vi "GSP_Main.vi"() -> ()   [LabVIEW 2015]
uses:
  Systems/Cam_Focus/CF_drivercontrol.ctl
  Systems/Wavelength/wavelength_driver_actions.ctl
  Silvermax/Monitor/handler_actions.ctl
  Log/LogItem.ctl
  Systems/Coll_Focus/coll_actions.ctl
  Systems/Grating_Translation/GTdriveractions.ctl
  Systems/Primary Filter/f1driveractions.ctl
  Systems/Secondary Filter/f2driveractions.ctl
  Systems/Slit/slitactions.ctl
  Systems/TCS_Link/TCSLINK_handler_actions.ctl
  GUI/GUI_states.ctl
  Systems/Cam_Focus/GSP_CF_Global.vi
  Systems/Wavelength/GSP_Wavelength_Global.vi
  Systems/SIcamera_Control/GPS_Drivers/GPS_Driver_Global.vi
  GUI/GSP_GUI_global.vi
  Systems/Primary Filter/GSP_F1_Global.vi
  Systems/Grating_Translation/GSP_GT_Global.vi
  Systems/Slit/GSP_SLIT_Global.vi
  Systems/Secondary Filter/GSP_F2_Global.vi
panel:
  out "TCS Connected":u16(ring)
  out "Camera Focus":u16(ring)
  out "Collimator Focus":u16(ring)
  out "Camera/Grating":u16(ring)
  out "Grating Selection":u16(ring)
  out "Mask Assembly":u16(ring)
  out "Secondary Filter":u16(ring)
  out "Primary Filter":u16(ring)
  out "Shutter Open":u16(ring)=2
  out "Camera flex target":dbl
  in  "Active?":bool=TRUE
  out "Right":i32
  out "Left":i32
  out "AnimatedControl":u16(ring)
  out "Instrument Connected":u16(ring)
  out "Last Error":errorcluster
  # "Flexure   Compensation"
  # "Wavelength Subpanel"
  # "Grating Subpanel"
  # "Slit Subpanel"
  # "Camera Subpanel"
  # "Collimator Subpanel"
  # "F2 Subpanel"
  # "F1 Subpanel"
  # "TCS Link\nSubpanel"
  # "Camera Control Subpanel"
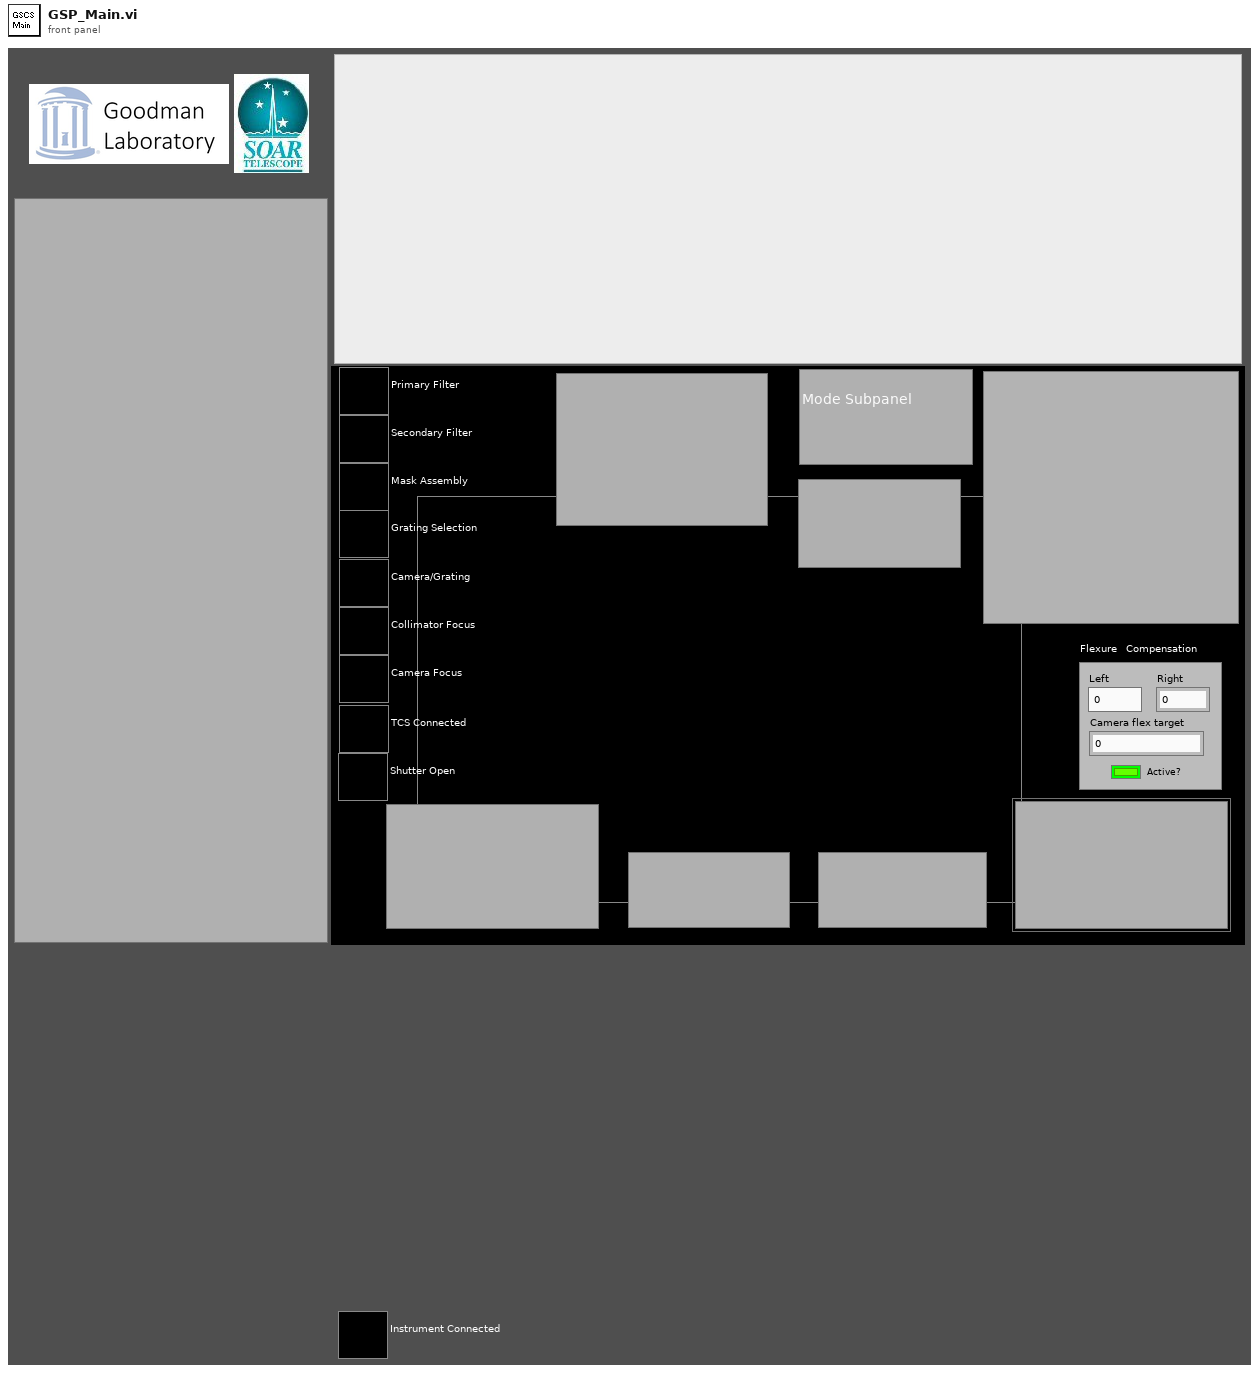
[diagram p1: front panel]
types:
  T1 = typedef "wavelength_driver_actions.ctl" = enum16{"Launch", "Flexure On", "Flexure Off", "Move", "Home", "Shutdown"}
  T2 = typedef "CF_drivercontrol.ctl" = enum16{"Launch", "Move", "Set Piezos", "Flexure On", "Flexure Off", "Home", "Shutdown"}
  T3 = typedef "handler_actions.ctl" = enum16{"Launch", "Shutdown All", "Shutdown"}
  T4 = enum16{"Launch", "Log", "Open", "Close", "Shutdown"}
  T5 = typedef "LogItem.ctl" = cluster{"error in (no error)":errorcluster, "Source":string, "Comment ":string}
  T6 = typedef "coll_actions.ctl" = enum16{"Launch", "Move", "Home", "Open Shutter", "Close Shutter", "Shutdown"}
  T7 = typedef "GTdriveractions.ctl" = enum16{"Launch", "INIT_CTL", "Move", "Home", "Shutdown"}
  T8 = typedef "f1driveractions.ctl" = enum16{"Launch", "INIT_CTL", "Home", "Move", "Shutdown"}
  T9 = typedef "f2driveractions.ctl" = enum16{"Launch", "INIT_CTL", "Home", "Move", "Shutdown"}
  T10 = typedef "slitactions.ctl" = enum16{"Launch", "INIT_CTL", "Restart", "Show", "Hide", "Home", "Move", "Rotate Only", "Shutdown"}
  T11 = typedef "TCSLINK_handler_actions.ctl" = enum16{"Launch", "Shutdown"}
  T12 = typedef "GUI_states.ctl" = enum16{"Logged Out", "Observer", "Operator", "Engineer"}
  T13 = cluster{"Primary Filter Names":string[], "Secondary Filter Names":string[], "Grating Names":string[], "Slit Mask Names":string[]}
  T14 = typedef "ThreadStates.ctl" = enum16{"Waiting", "Scripting", "Uninitialized", "Error"}
  T15 = cluster{"GT Thread state":T14, "Slit Thread State":T14, "F1 Thread State":T14, "F2 Thread State":T14, "Coll Thread State":T14, "CF Thread State":T14, "Wavelength Thread State":T14}
  T16 = cluster{"Grating#":i32, "Slit#":i32, "Primary Filter#":i32, "Secondary Filter#":i32, "Coll Position":i32, "Camera Focus":i32, "Camera Angle":dbl, "Grating Angle":dbl, "Coll Temp":dbl, "CF Temp\n":dbl, "Camera Target":dbl, "Grating Target":dbl, "WAVMODE":string, "Slit Hidden??":bool}
  T17 = cluster{"Init Primary Filter":bool, "Init Secondary Filter":bool, "Init Coll Focus":bool, "Init Camera Focus":bool, "Init Slit":bool, "Init Grating Trans":bool, "Init Wavelength":bool}
  T18 = cluster{"Primary Filter Names":string[], "Secondary Filter Names":string[], "Grating Names":string[], "Slit Mask Names":string[], "Standard Observing Modes":string[]}
  T19 = cluster{"F1_Name":string, "F2_Name":string, "Slit Name":string, "Grating Name":string, "Camera Target":dbl, "Grating Target":dbl, "Coll Position":i32, "Camera Focus":i32, string, string, string, string, "Flexure Active":bool, i32}
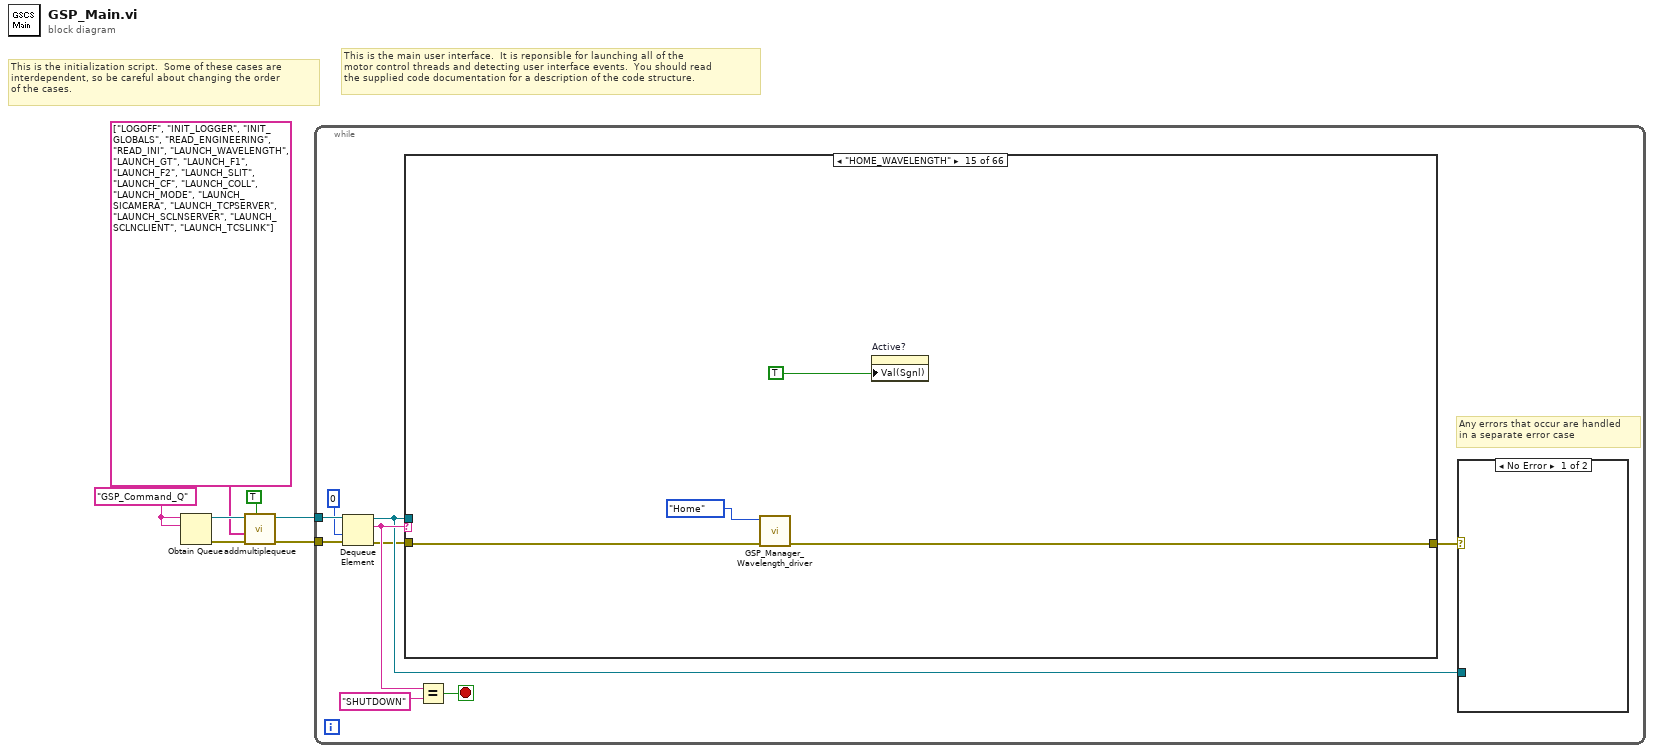
[diagram p0: block diagram]
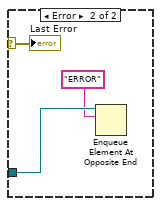
[diagram p2: hidden frame]
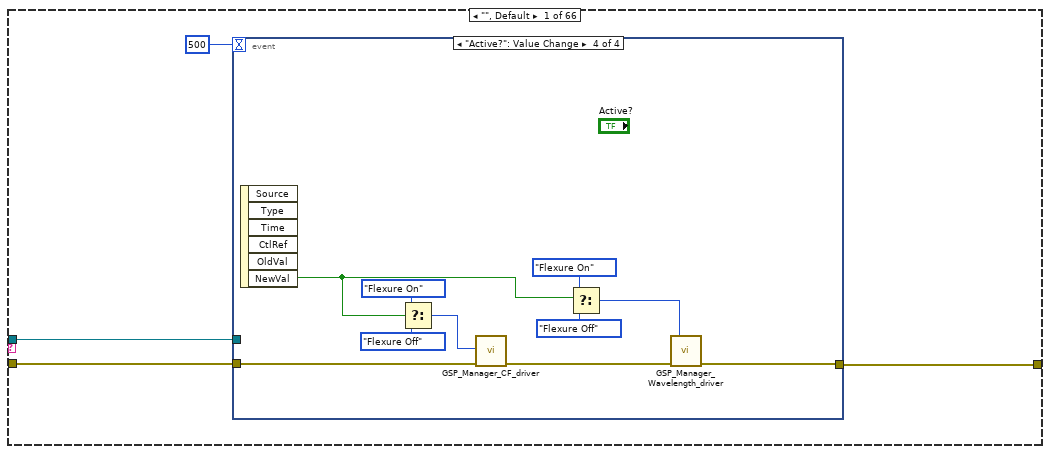
[diagram p3: hidden frame]
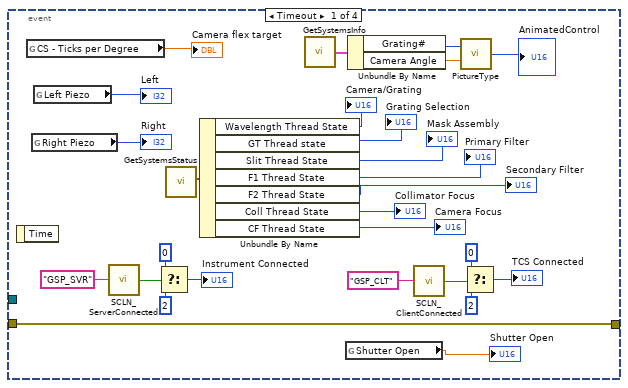
[diagram p4: hidden frame]
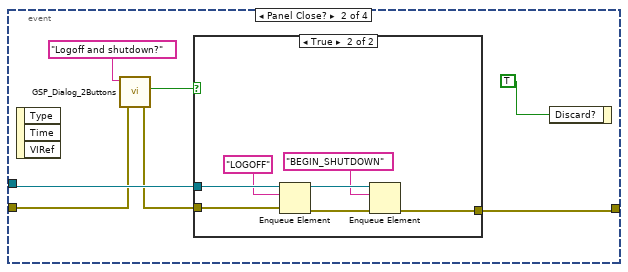
[diagram p5: hidden frame]
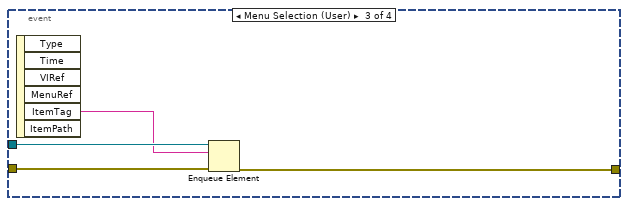
[diagram p7: hidden frame]
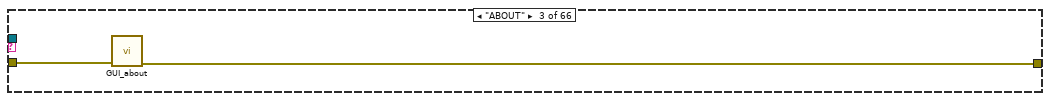
[diagram p9: hidden frame]
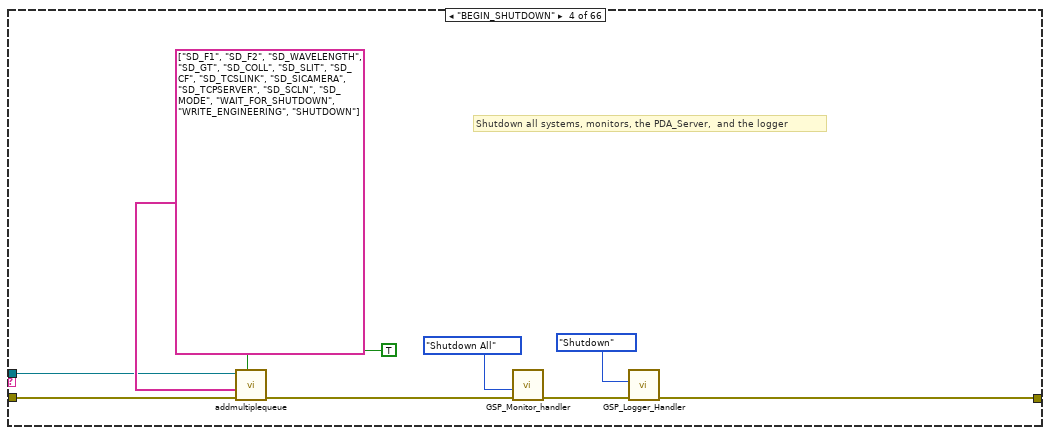
[diagram p10: hidden frame]
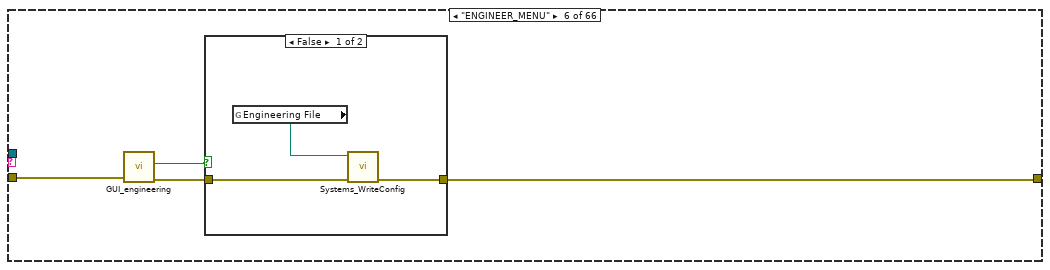
[diagram p12: hidden frame]
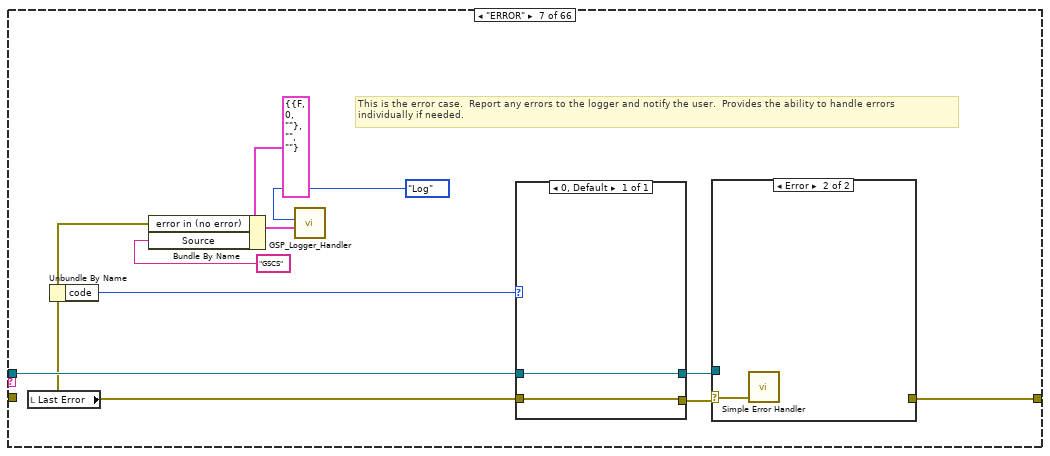
[diagram p14: hidden frame]
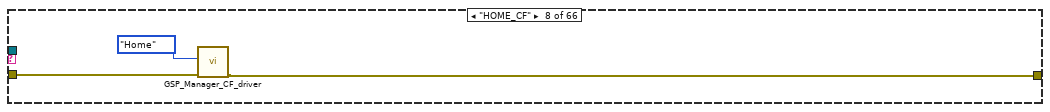
[diagram p16: hidden frame]
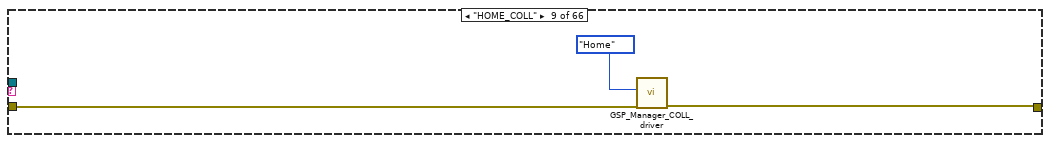
[diagram p17: hidden frame]
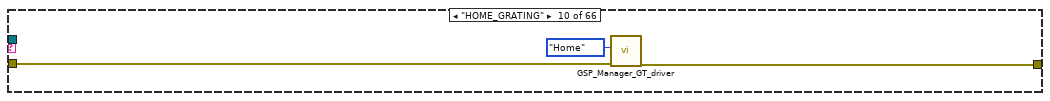
[diagram p18: hidden frame]
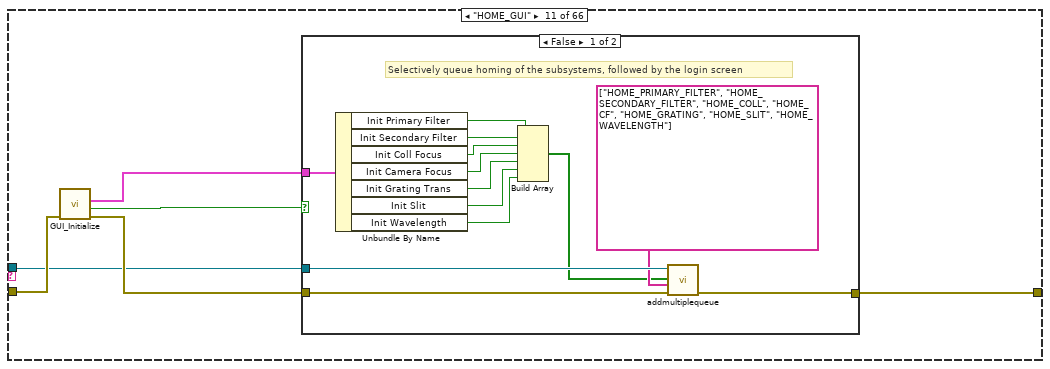
[diagram p19: hidden frame]
diagram:
  w7 = "GSP_Command_Q" ("name (unnamed)")
  # "This is the initialization script.  Some of these cases are\ninterdependent, so be careful about changing the order\nof the cases."
  # "This is the main user interface.  It is reponsible for launching all of the \nmotor control threads and detecting user interface events.  You should read \nthe supplied code documentation for a description of the code structure."
  n1 = Obtain Queue(name (unnamed)=w7, element data type=w7) -> (queue out=w3:refnum<queue>, error out=w5:errorcluster)  [unwired: 3 in, 1 out]
  n2 = call "addmultiplequeue.vi"("Add All (false)"=TRUE, "error in (no error)"=w5, "Strings to Add"=string[] ["LOGOFF", "INIT_LOGGER", "INIT_GLOBALS", "READ_ENGINEERING", "READ_INI", "LAUNCH_WAVELENGTH", "LAUNCH_GT", "LAUNCH_F1", "LAUNCH_F2", "LAUNCH_SLIT", "LAUNCH_CF", "LAUNCH_COLL", "LAUNCH_MODE", "LAUNCH_SICAMERA", "LAUNCH_TCPSERVER", "LAUNCH_SCLNSERVER", "LAUNCH_SCLNCLIENT", "LAUNCH_TCSLINK"], "queue"=w3) -> ("error out"=w1:errorcluster, "queue out"=w6:refnum<queue>)  [unwired: 3 in]
  n3 = while {
    tunnel: w1 -> [w15]
    tunnel: w6 -> [w16]
    stop <- w12 stop-if-true
    # "Any errors that occur are handled\nin a separate error case"
    n4 = Dequeue Element(queue=w16, timeout in ms (-1)=0, error in (no error)=w15) -> (queue out=w11:refnum<queue>, element=w14:string, error out=w9:errorcluster)  [unwired: 1 out]
    n5 = case shown="\"HOME_WAVELENGTH\"" w14 {
      tunnel: w11 -> [w23 _ _ w87 _ _ w108 _ _ _ w126 _ _ _ _ _ _ _ _ _ _ _ _ _ _ _ _ _ _ _ _ _ w267 w280 _ _ _ _ _ _ _ _ _ _ _ _ _ _ _ _ _ _ _ _ _ _ _ _ _ _ w425 _ _ _ _ _]
      tunnel: w9 -> [w22 w80 w82 w89 w92 w96 _ w117 w120 w123 w129 w146 w149 w152 w156 w165 w182 w197 w203 w208 w213 w218 w222 w228 w232 w237 w242 w248 w251 w254 w257 w258 w270 w283 w302 w308 w312 w319 w325 w332 w338 w344 w350 w354 w358 w365 w383 w386 w389 w391 w395 w398 w401 w404 w407 w409 w413 w416 _ w423 _ w432 w441 w445 w448 w449]
      tunnel: [w21 w80 w81 w83 w92 w93 w106 w115 w119 w122 w125 w145 w148 w151 w154 w158 w175 w196 w200 w204 w209 w215 w219 w225 w229 w235 w243 w246 w249 w252 w255 w261 w268 w279 w297 w303 w311 w315 w323 w328 w335 w341 w347 w352 w357 w365 w382 w385 w388 w392 w394 w397 w400 w403 w406 w408 w412 w415 _ w421 w424 w428 w436 w444 w447 _] -> w8
      frame "", Default {
        n6 = event shown="[3] \"Active?\": Value Change" {
          selector: _ -> [_ _ _ _]
          dyn-events: _ -> [_ _ _ _]
          timeout: 500 -> [_ _ _ _]
          tunnel: w23 -> [_ w56 w69 _]
          tunnel: [w43 w55 w66 w74] -> w21
          tunnel: w22 -> [w43 w53 w67 w79]
          event Timeout {
            n7 = event-data() -> ()  [unwired: 1 in, 1 out]
            n8 = global read "GSP_Wavelength_Global.vi" "CS - Ticks per Degree"() -> (→"Camera flex target":dbl)
            n9 = global read "GSP_CF_Global.vi" "Right Piezo"() -> (→"Right":i32)
            n10 = global read "GSP_CF_Global.vi" "Left Piezo"() -> (→"Left":i32)
            n11 = call "SCLN_ServerConnected.vi"("Server Name"="GSP_SVR" ("String")) -> ("Connected"=w31:bool)
            n12 = Select(t=u16 0, s=w31, f=u16 2) -> (s? t:f=→"Instrument Connected":u16)
            n13 = call "GetSystemsStatus.vi"() -> ("Thread States"=w42:T15)  [unwired: 4 in, 3 out]
            n14 = Unbundle By Name(w42) -> ("Wavelength Thread State"=→"Camera/Grating":T14, "GT Thread state"=→"Grating Selection":T14, "Slit Thread State"=→"Mask Assembly":T14, "F1 Thread State"=→"Primary Filter":T14, "F2 Thread State"=→"Secondary Filter":T14, "Coll Thread State"=→"Collimator Focus":T14, "CF Thread State"=→"Camera Focus":T14)
            n15 = call "GetSystemsInfo.vi"() -> ("Pos Info"=w47:T16)
            n16 = global read "GPS_Driver_Global.vi" "Shutter Open"() -> (→"Shutter Open":dbl)
            n17 = Unbundle By Name(w47) -> ("Grating#"=w46:i32, "Camera Angle"=w45:dbl)
            n18 = call "SCLN_ClientConnected.vi"("Server Name"="GSP_CLT" ("String")) -> ("Connected"=w27:bool)
            n19 = call "PictureType.vi"("Camera Angle"=w45, "Grating#"=w46) -> ("GS_picture_tab"=→"AnimatedControl":u16)
            n20 = Select(t=u16 0, s=w27, f=u16 2) -> (s? t:f=→"TCS Connected":u16)
          }
          event Panel Close? {
            n21 = event-data() -> ()  [unwired: 1 in, 3 out]
            n22 = call "GSP_Dialog_2Buttons.vi"("error in (no error)"=w53, "Message"="Logoff and shutdown?" ("message")) -> ("error out"=w52:errorcluster, "OK Button?"=w51:bool)  [unwired: 4 in]
            n23 = case shown="True" w51 {
              tunnel: w52 -> [w58 w64]
              tunnel: w56 -> [_ w65]
              tunnel: [w58 w61] -> w55
              frame False {
              }
              frame True {
                n24 = Enqueue Element(queue=w65, element="LOGOFF", error in (no error)=w64) -> (queue out=w63:refnum<queue>, error out=w62:errorcluster)  [unwired: 1 in, 1 out]
                n25 = Enqueue Element(queue=w63, element="BEGIN_SHUTDOWN", error in (no error)=w62) -> (error out=w61:errorcluster)  [unwired: 1 in, 2 out]
              }
            }
            n26 = event-data("Discard?"=TRUE) -> ()  [unwired: 1 in, 1 out]
          }
          event Menu Selection (User) {
            n27 = event-data() -> ("ItemTag"=w68:string)  [unwired: 1 in, 5 out]
            n28 = Enqueue Element(queue=w69, element=w68, error in (no error)=w67) -> (error out=w66:errorcluster)  [unwired: 1 in, 2 out]
          }
          event "Active?": Value Change {
            n29 = event-data() -> ("NewVal"=w71:bool)  [unwired: 1 in, 5 out]
            n30 = Select(t=CF_drivercontrol."Flexure On" ("Action"), s=w71, f=CF_drivercontrol."Flexure Off" ("Action")) -> (s? t:f=w76:T2)
            n31 = call "GSP_Manager_CF_driver.vi"("error in (no error)"=w79, "Action"=w76) -> ("error out"=w75:errorcluster)  [unwired: 5 in, 1 out]
            n32 = Select(t=wavelength_driver_actions."Flexure On" ("Action"), s=w71, f=wavelength_driver_actions."Flexure Off" ("Action")) -> (s? t:f=w70:T1)
            n33 = call "GSP_Manager_Wavelength_driver.vi"("error in (no error)"=w75, "Action"=w70) -> ("error out"=w74:errorcluster)  [unwired: 4 in, 1 out]
          }
        }
      }
      frame "REFRESH_CONTROLS" {
        # "This case addresses a bug in remote panel builds.  Forces\na refresh of the control.disabled property for controls on the remote\npanel"
      }
      frame "ABOUT" {
        n34 = call "GUI_about.vi"("error in (no error)"=w82) -> ("error out"=w81:errorcluster)  [unwired: 6 in]
      }
      frame "BEGIN_SHUTDOWN" {
        # "Shutdown all systems, monitors, the PDA_Server,  and the logger"
        n35 = call "addmultiplequeue.vi"("Add All (false)"=TRUE, "error in (no error)"=w89, "Strings to Add"=string[] ["SD_F1", "SD_F2", "SD_WAVELENGTH", "SD_GT", "SD_COLL", "SD_SLIT", "SD_CF", "SD_TCSLINK", "SD_SICAMERA", "SD_TCPSERVER", "SD_SCLN", "SD_MODE", "WAIT_FOR_SHUTDOWN", "WRITE_ENGINEERING", "SHUTDOWN"], "queue"=w87) -> ("error out"=w88:errorcluster)  [unwired: 3 in, 1 out]
        n36 = call "GSP_Monitor_handler.vi"("error in (no error)"=w88, "Action"=handler_actions."Shutdown All") -> ("error out"=w86:errorcluster)  [unwired: 5 in, 1 out]
        n37 = call "GSP_Logger_Handler.vi"("error in (no error)"=w86, "Actions"=T4."Shutdown") -> ("error out"=w83:errorcluster)  [unwired: 5 in]
      }
      frame "DOCUMENTATION" {
      }
      frame "ENGINEER_MENU" {
        n38 = call "GUI_engineering.vi"("error in (no error)"=w96) -> ("error out"=w95:errorcluster, "Canceled?"=w94:bool)  [unwired: 5 in]
        n39 = case shown="False" w94 {
          tunnel: w95 -> [w99 w100]
          tunnel: [w98 w100] -> w93
          frame False {
            n40 = global read "GSP_GUI_global.vi" "Engineering File"() -> (w97:path)
            n41 = call "Systems_WriteConfig.vi"("error in (no error)"=w99, "configuration file path"=w97) -> ("error out"=w98:errorcluster)  [unwired: 5 in]
          }
          frame True {
          }
        }
      }
      frame "ERROR" {
        # "This is the error case.  Report any errors to the logger and notify the user.  Provides the ability to handle errors\nindividually if needed."
        n42 = local read "Last Error"() -> (w102:errorcluster)
        n43 = Unbundle By Name(w102) -> ("code"=w110:i32)
        n44 = Bundle By Name(cluster=T5 {"error in (no error)"={"status"=FALSE, "code"=0, "source"=""}, "Source"="", "Comment "=""} ("Log"), "error in (no error)"=w102, "Source"="GSCS") -> (w103:T5)
        n45 = call "GSP_Logger_Handler.vi"("Log"=w103, "Actions"=T4."Log") -> ()  [unwired: 5 in, 1 out]
        n46 = case shown="0, Default" w110 {
          tunnel: w102 -> [w114]
          tunnel: [w114] -> w109
          tunnel: w108 -> [w113]
          tunnel: [w113] -> w107
          frame 0, Default {
          }
        }
        n47 = case shown="Error" w109 {
          selector: w109 -> [w111 w112]
          tunnel: [w111 _] -> w106
          tunnel: w107 -> [_ _]
          frame No Error {
          }
          frame Error {
            n48 = call <vilib>:"Simple Error Handler.vi"("error in (no error)"=w112) -> ()  [unwired: 4 in, 5 out]
          }
        }
      }
      frame "HOME_CF" {
        n49 = call "GSP_Manager_CF_driver.vi"("error in (no error)"=w117, "Action"=CF_drivercontrol."Home") -> ("error out"=w115:errorcluster)  [unwired: 5 in, 1 out]
      }
      frame "HOME_COLL" {
        n50 = call "GSP_Manager_COLL_driver.vi"("error in (no error)"=w120, "Action"=coll_actions."Home") -> ("error out"=w119:errorcluster)  [unwired: 4 in, 1 out]
      }
      frame "HOME_GRATING" {
        n51 = call "GSP_Manager_GT_driver.vi"("error in (no error)"=w123, "Action"=GTdriveractions."Home") -> ("error out"=w122:errorcluster)  [unwired: 4 in, 1 out]
      }
      frame "HOME_GUI" {
        n52 = call "GUI_Initialize.vi"("error in (no error)"=w129) -> ("error out"=w128:errorcluster, "Canceled?"=w127:bool, "Initialize Out"=w124:T17)  [unwired: 4 in]
        n53 = case shown="False" w127 {
          tunnel: w128 -> [w141 w143]
          tunnel: w126 -> [w140 _]
          tunnel: [w130 w143] -> w125
          tunnel: w124 -> [w142 _]
          frame False {
            # "Selectively queue homing of the subsystems, followed by the login screen"
            n54 = Unbundle By Name(w142) -> ("Init Primary Filter"=w137:bool, "Init Secondary Filter"=w131:bool, "Init Coll Focus"=w136:bool, "Init Camera Focus"=w135:bool, "Init Grating Trans"=w134:bool, "Init Slit"=w133:bool, "Init Wavelength"=w132:bool)
            n55 = Build Array(w137, w131, w136, w135, w134, w133, w132) -> (w138:bool[])
            n56 = call "addmultiplequeue.vi"("error in (no error)"=w141, "Strings to Add"=string[] ["HOME_PRIMARY_FILTER", "HOME_SECONDARY_FILTER", "HOME_COLL", "HOME_CF", "HOME_GRATING", "HOME_SLIT", "HOME_WAVELENGTH"], "Add String?"=w138, "queue"=w140) -> ("error out"=w130:errorcluster)  [unwired: 3 in, 1 out]
          }
          frame True {
          }
        }
      }
      frame "HOME_PRIMARY_FILTER" {
        n57 = call "GSP_Manager_F1_driver.vi"("error in (no error)"=w146, "Action"=f1driveractions."Home") -> ("error out"=w145:errorcluster)  [unwired: 4 in, 1 out]
      }
      frame "HOME_SECONDARY_FILTER" {
        n58 = call "GSP_Manager_F2_driver.vi"("error in (no error)"=w149, "Action"=f2driveractions."Home") -> ("error out"=w148:errorcluster)  [unwired: 4 in, 1 out]
      }
      frame "HOME_SLIT" {
        n59 = call "GSP_Manager_Slit_driver.vi"("error in (no error)"=w152, "Action"=slitactions."Home") -> ("error out"=w151:errorcluster)  [unwired: 4 in, 1 out]
      }
      frame "HOME_WAVELENGTH" {
        n60 = call "GSP_Manager_Wavelength_driver.vi"("error in (no error)"=w156, "Action"=wavelength_driver_actions."Home") -> ("error out"=w154:errorcluster)  [unwired: 4 in, 1 out]
        n61 = property on="Active?" class="Bool (strict)"("Val(Sgnl)"=TRUE) -> ()  [unwired: 2 in, 2 out]
      }
      frame "INIT_CONTROLS" {
        n62 = call "GSP_Manager_F1_driver.vi"("error in (no error)"=w165, "Action"=f1driveractions."INIT_CTL") -> ("error out"=w163:errorcluster)  [unwired: 4 in, 1 out]
        n63 = call "GSP_Manager_F2_driver.vi"("error in (no error)"=w163, "Action"=f2driveractions."INIT_CTL") -> ("error out"=w161:errorcluster)  [unwired: 4 in, 1 out]
        n64 = call "GSP_Manager_Slit_driver.vi"("error in (no error)"=w161, "Action"=slitactions."INIT_CTL") -> ("error out"=w159:errorcluster)  [unwired: 4 in, 1 out]
        n65 = call "GSP_Manager_GT_driver.vi"("error in (no error)"=w159, "Action"=GTdriveractions."INIT_CTL") -> ("error out"=w158:errorcluster)  [unwired: 4 in, 1 out]
      }
      frame "INIT_GLOBALS" {
        w169 = path "\\\\SHERMAN-PC\\Config"
        # "Detects wether this is a build or development"
        # "Initialize all of the global file paths, detecting wether you are in a build\nor development environment."
        # "Initialize the Silvermax serial port and reboot all of the motors using the group ID"
        n66 = call "gsp_silvermax_setup.vi"("error in (no error)"=w182, "Timeout (1000 ms)"=u32 100, "VISA resource name"=refnum<visa-resource-name> "COM1") -> ("error out"=w175:errorcluster)  [unwired: 4 in]
        n67 = Current VI's Path() -> (path=w187:path)
        n68 = Strip Path(path=w187) -> (stripped path=w166:path, name=w167:string)
        n69 = local write "Active?"(FALSE) -> ()
        n70 = Match Pattern(string=w167, regular expression=".exe") -> (offset past match=w191:i32)  [unwired: 1 in, 3 out]
        n71 = case shown="0, Default" w191 {
          tunnel: w166 -> [w194 w195]
          tunnel: [w194 w195] -> w171
          tunnel: w167 -> [_ _]
          frame 0, Default {
          }
          frame -1 {
          }
        }
        n72 = Build Path(base path=w169, name or relative path="observing_modes.ini") -> (appended path=w173:path)
        n73 = Build Path(base path=w169, name or relative path="engineering.ini") -> (appended path=w193:path)
        n74 = global write "GSP_GUI_global.vi" "Standard Observing Modes File"(w173) -> ()
        n75 = global write "GSP_GUI_global.vi" "Engineering File"(w193) -> ()
        n76 = Build Path(base path=w169, name or relative path="masks.ini") -> (appended path=w178:path)
        n77 = Build Path(base path=w169, name or relative path="filters.ini") -> (appended path=w179:path)
        n78 = Build Path(base path=w169, name or relative path="gratings.ini") -> (appended path=w185:path)
        n79 = Build Path(base path=w169, name or relative path="masterconfig.ini") -> (appended path=w170:path)
        n80 = Build Path(base path=w171, name or relative path="users.ini") -> (appended path=w177:path)
        n81 = Build Path(base path=w171, name or relative path="Users") -> (appended path=w189:path)
        n82 = global write "GSP_GUI_global.vi" "Configuration File"(w170) -> ()
        n83 = global write "GSP_GUI_global.vi" "UserFile"(w177) -> ()
        n84 = global write "GSP_GUI_global.vi" "Filter File"(w179) -> ()
        n85 = global write "GSP_GUI_global.vi" "Slit File"(w178) -> ()
        n86 = global write "GSP_GUI_global.vi" "Grating File"(w185) -> ()
        n87 = global write "GSP_GUI_global.vi" "UserPath"(w189) -> ()
      }
      frame "INIT_LOGGER" {
        n88 = call "GSP_Logger_Handler.vi"("error in (no error)"=w197, "Actions"=T4."Launch") -> ("error out"=w196:errorcluster)  [unwired: 5 in]
      }
      frame "LAUNCH_WAVELENGTH" {
        # "Motor manager threads are launched by supplying control references to the controls that threads will update.  This case launches\nthe collimator thread.  Events on the controls are still detected in the main interface and relayed to the manager threads by using the\ninterface below with the appropriate action."
        n89 = call "GSP_Manager_Wavelength_driver.vi"("error in (no error)"=w203, "Action"=wavelength_driver_actions."Launch") -> ("error out"=w201:errorcluster, "VI reference (launch only)"=w199:refnum<vi>)  [unwired: 4 in]
        n90 = invoke on="Camera/Grating Angles" class="SubPanel" method="Insert VI"(error in=w201, "VI Ref"=w199) -> (error out=w200:errorcluster)  [unwired: 2 in, 3 out]
      }
      frame "LAUNCH_COLL" {
        n91 = call "GSP_Manager_COLL_driver.vi"("error in (no error)"=w208, "Action"=coll_actions."Launch") -> ("error out"=w206:errorcluster, "reference out (launch only)"=w205:refnum<vi>)  [unwired: 4 in]
        n92 = invoke on="Collimator Subpanel" class="SubPanel" method="Insert VI"(error in=w206, "VI Ref"=w205) -> (error out=w204:errorcluster)  [unwired: 2 in, 3 out]
      }
      frame "LAUNCH_CF" {
        n93 = call "GSP_Manager_CF_driver.vi"("error in (no error)"=w213, "Action"=CF_drivercontrol."Launch") -> ("error out"=w211:errorcluster, "reference out (launch only)"=w210:refnum<vi>)  [unwired: 5 in]
        n94 = invoke on="Camera Subpanel" class="SubPanel" method="Insert VI"(error in=w211, "VI Ref"=w210) -> (error out=w209:errorcluster)  [unwired: 2 in, 3 out]
      }
      frame "LAUNCH_F1" {
        n95 = call "GSP_Manager_F1_driver.vi"("error in (no error)"=w218, "Action"=f1driveractions."Launch") -> ("error out"=w217:errorcluster, "reference out (launch only)"=w216:refnum<vi>)  [unwired: 4 in]
        n96 = invoke on="F1 Subpanel" class="SubPanel" method="Insert VI"(error in=w217, "VI Ref"=w216) -> (error out=w215:errorcluster)  [unwired: 2 in, 3 out]
      }
      frame "LAUNCH_F2" {
        n97 = call "GSP_Manager_F2_driver.vi"("error in (no error)"=w222, "Action"=f2driveractions."Launch") -> ("error out"=w221:errorcluster, "reference out (launch only)"=w220:refnum<vi>)  [unwired: 4 in]
        n98 = invoke on="F1 Subpanel" class="SubPanel" method="Insert VI"(error in=w221, "VI Ref"=w220) -> (error out=w219:errorcluster)  [unwired: 2 in, 3 out]
      }
      frame "LAUNCH_GT" {
        n99 = call "GSP_Manager_GT_driver.vi"("error in (no error)"=w228, "Action"=GTdriveractions."Launch") -> ("error out"=w227:errorcluster, "reference out (launch only)"=w226:refnum<vi>)  [unwired: 4 in]
        n100 = invoke on="Grating Subpanel" class="SubPanel" method="Insert VI"(error in=w227, "VI Ref"=w226) -> (error out=w225:errorcluster)  [unwired: 2 in, 3 out]
      }
      frame "LAUNCH_SLIT" {
        n101 = call "GSP_Manager_Slit_driver.vi"("error in (no error)"=w232, "Action"=slitactions."Launch") -> ("error out"=w231:errorcluster, "reference out (launch only)"=w230:refnum<vi>)  [unwired: 4 in]
        n102 = invoke on="Slit Subpanel" class="SubPanel" method="Insert VI"(error in=w231, "VI Ref"=w230) -> (error out=w229:errorcluster)  [unwired: 2 in, 3 out]
      }
      frame "LAUNCH_TCSLINK" {
        n103 = call "GSP_Manager_TCSLINK_handler.vi"("error in (no error)"=w237, "Actions"=TCSLINK_handler_actions."Launch") -> ("error out"=w236:errorcluster, "reference out (launch only)"=w234:refnum<vi>)  [unwired: 4 in]
        n104 = invoke on="TCS_SubPanel" class="SubPanel" method="Insert VI"(error in=w236, "VI Ref"=w234) -> (error out=w235:errorcluster)  [unwired: 2 in, 3 out]
      }
      frame "LAUNCH_SICAMERA" {
        n105 = call "SIcamera_Driver.vi"("error in (no error)"=w242, "Action"=enum16{"Launch", "Shutdown"}."Launch") -> ("error out"=w239:errorcluster, "reference out (launch only)"=w240:refnum<vi>)  [unwired: 4 in]
        n106 = invoke on="SIcamera Control Panel" class="SubPanel" method="Insert VI"(error in=w239, "VI Ref"=w240) -> (error out=w243:errorcluster)  [unwired: 2 in, 3 out]
      }
      frame "LAUNCH_MODE" {
        n107 = call "Mode_driver.vi"("error in (no error)"=w248, "Action"=enum16{"Launch", "Shutdown"}."Launch") -> ("error out"=w247:errorcluster, "reference out (launch only)"=w244:refnum<vi>)  [unwired: 4 in]
        n108 = invoke on="Mode Subpanel" class="SubPanel" method="Insert VI"(error in=w247, "VI Ref"=w244) -> (error out=w246:errorcluster)  [unwired: 2 in, 3 out]
      }
      frame "LAUNCH_TCPSERVER" {
        n109 = call "TCPServer_driver.vi"("error in (no error)"=w251, "Action"=enum16{"Launch", "Shutdown"}."Launch") -> ("error out"=w249:errorcluster)  [unwired: 5 in]
      }
      frame "LAUNCH_SCLNSERVER" {
        n110 = call "GSP_Manager_SCLNServer_Handler.vi"("error in (no error)"=w254, "Actions"=TCSLINK_handler_actions."Launch") -> ("error out"=w252:errorcluster)  [unwired: 4 in, 1 out]
      }
      frame "LAUNCH_SCLNCLIENT" {
        n111 = call "GSP_Manager_SCLNClient_Handler.vi"("error in (no error)"=w257, "Actions"=TCSLINK_handler_actions."Launch") -> ("error out"=w255:errorcluster)  [unwired: 4 in, 1 out]
      }
      frame "LOGOFF" {
        # "Set the interface to a Logged Off mode"
        n112 = global write "GSP_GUI_global.vi" "Current User"("NO USER" ("Current User")) -> ()
        n113 = global write "GSP_GUI_global.vi" "User Type"(i8 0 ("User Type")) -> ()
        n114 = Current VI's Menubar() -> (w263:refnum<k9>)
        n115 = call "GSP_setmenu.vi"("error in (no error)"=w258, "GUI States"=GUI_states."Logged Out", "menubar"=w263) -> ("error out"=w261:errorcluster)  [unwired: 4 in]
      }
      frame "LOGON" {
        n116 = global read "GSP_GUI_global.vi" "UserFile"() -> (w264:path)
        n117 = call "GSP_GUI_user.vi"("error in"=w270, "User File"=w264) -> ("error out"=w269:errorcluster, "User Type"=w265:T12, "Canceled?"=w266:bool)  [unwired: 3 in]
        n118 = case shown="False" w266 {
          tunnel: w269 -> [w271 w275]
          tunnel: [w272 w275] -> w268
          tunnel: w267 -> [_ _]
          tunnel: w265 -> [w273 _]
          frame False {
            n119 = Current VI's Menubar() -> (w274:refnum<k9>)
            n120 = call "GSP_setmenu.vi"("error in (no error)"=w271, "GUI States"=w273, "menubar"=w274) -> ("error out"=w272:errorcluster)  [unwired: 4 in]
          }
          frame True {
          }
        }
      }
      frame "MASTER_CONFIG_GUI" {
        # "Open the Configuration Manager. If the user makes changes to the configuration file, reload the file and update the controls."
        n121 = global read "GSP_GUI_global.vi" "Filter File"() -> (w277:path)
        n122 = global read "GSP_GUI_global.vi" "Slit File"() -> (w276:path)
        n123 = global read "GSP_GUI_global.vi" "Grating File"() -> (w278:path)
        n124 = call "GSP_MasterConfiguration.vi"("error in (no error)"=w283, "Slit File"=w276, "Filter File"=w277, "grating file"=w278) -> ("error out"=w281:errorcluster, "Changes Made?"=w282:bool)  [unwired: 3 in]
        n125 = case shown="True" w282 {
          tunnel: w281 -> [w284 w293]
          tunnel: w280 -> [_ w294]
          tunnel: [w284 w296] -> w279
          frame False {
          }
          frame True {
            n126 = global read "GSP_GUI_global.vi" "Secondary Filter Names"() -> (w288:string[])
            n127 = global read "GSP_GUI_global.vi" "Primary Filter Names"() -> (w289:string[])
            n128 = global read "GSP_GUI_global.vi" "Grating Names"() -> (w287:string[])
            n129 = global read "GSP_GUI_global.vi" "Slit Mask Names"() -> (w286:string[])
            n130 = Bundle By Name(cluster=T13 {"Primary Filter Names"=[], "Secondary Filter Names"=[], "Grating Names"=[], "Slit Mask Names"=[]} ("Present Configuration"), "Primary Filter Names"=w289, "Secondary Filter Names"=w288, "Grating Names"=w287, "Slit Mask Names"=w286) -> (w285:T13)
            n131 = global read "GSP_GUI_global.vi" "Configuration File"() -> (w291:path)
            n132 = call "Write_Master_Config.vi"("error in (no error)"=w293, "Present Configuration"=w285, "configuration file path"=w291) -> ("error out"=w292:errorcluster)  [unwired: 4 in]
            n133 = Enqueue Element(queue=w294, element="INIT_CONTROLS", error in (no error)=w292) -> (error out=w296:errorcluster)  [unwired: 1 in, 2 out]
          }
        }
      }
      frame "MONITOR_COLL" {
        w299 = u16 1 items=["External", "Internal"] ("Mode")
        # "This is an example of how to launch a motor monitor and open the front panel"
        n134 = call "GSP_Monitor_handler.vi"("Mode"=w299, "error in (no error)"=w302, "Action"=handler_actions."Launch", "Motor#"=u8 40, "Monitor Name"="Collimator Focus") -> ("error out"=w297:errorcluster)  [unwired: 2 in, 1 out]
      }
      frame "MONITOR_CF" {
        w305 = u16 1 items=["External", "Internal"] ("Mode")
        # "This is an example of how to launch a motor monitor and open the front panel"
        n135 = call "GSP_Monitor_handler.vi"("Mode"=w305, "error in (no error)"=w308, "Action"=handler_actions."Launch", "Motor#"=u8 46, "Monitor Name"="Camera Focus") -> ("error out"=w303:errorcluster)  [unwired: 2 in, 1 out]
      }
      frame "MONITOR_CS" {
        w310 = u16 0 items=["External", "Internal"] ("Mode")
        n136 = call "GSP_Monitor_handler.vi"("Mode"=w310, "error in (no error)"=w312, "Action"=handler_actions."Launch", "Motor#"=u8 45, "Monitor Name"="Camera Stage") -> ("error out"=w311:errorcluster)  [unwired: 2 in, 1 out]
      }
      frame "MONITOR_F1" {
        w317 = u16 1 items=["External", "Internal"] ("Mode")
        n137 = call "GSP_Monitor_handler.vi"("Mode"=w317, "error in (no error)"=w319, "Action"=handler_actions."Launch", "Motor#"=u8 47, "Monitor Name"="Primary Filter Wheel") -> ("error out"=w315:errorcluster)  [unwired: 2 in, 1 out]
      }
      frame "MONITOR_F2" {
        w322 = u16 1 items=["External", "Internal"] ("Mode")
        n138 = call "GSP_Monitor_handler.vi"("Mode"=w322, "error in (no error)"=w325, "Action"=handler_actions."Launch", "Motor#"=u8 48, "Monitor Name"="Secondary Filter Wheel") -> ("error out"=w323:errorcluster)  [unwired: 2 in, 1 out]
      }
      frame "MONITOR_GS" {
        w329 = u16 0 items=["External", "Internal"] ("Mode")
        n139 = call "GSP_Monitor_handler.vi"("Mode"=w329, "error in (no error)"=w332, "Action"=handler_actions."Launch", "Motor#"=u8 43, "Monitor Name"="Grating Stage") -> ("error out"=w328:errorcluster)  [unwired: 2 in, 1 out]
      }
      frame "MONITOR_GT" {
        w334 = u16 1 items=["External", "Internal"] ("Mode")
        n140 = call "GSP_Monitor_handler.vi"("Mode"=w334, "error in (no error)"=w338, "Action"=handler_actions."Launch", "Motor#"=u8 44, "Monitor Name"="Grating Translation") -> ("error out"=w335:errorcluster)  [unwired: 2 in, 1 out]
      }
      frame "MONITOR_SLIT_ROT" {
        w339 = u16 1 items=["External", "Internal"] ("Mode")
        n141 = call "GSP_Monitor_handler.vi"("Mode"=w339, "error in (no error)"=w344, "Action"=handler_actions."Launch", "Motor#"=u8 41, "Monitor Name"="Slit Rotation") -> ("error out"=w341:errorcluster)  [unwired: 2 in, 1 out]
      }
      frame "MONITOR_SLIT_TRANS" {
        w346 = u16 1 items=["External", "Internal"] ("Mode")
        n142 = call "GSP_Monitor_handler.vi"("Mode"=w346, "error in (no error)"=w350, "Action"=handler_actions."Launch", "Motor#"=u8 42, "Monitor Name"="Slit Translation") -> ("error out"=w347:errorcluster)  [unwired: 2 in, 1 out]
      }
      frame "READ_ENGINEERING" {
        # "Read the engineering file.  This loads all of the motor manager global variables with the appropriate values."
        n143 = global read "GSP_GUI_global.vi" "Engineering File"() -> (w353:path)
        n144 = call "Systems_ReadConfig.vi"("error in (no error)"=w354, "configuration file path"=w353) -> ("error out"=w352:errorcluster, "All Found?"=w351:bool)  [unwired: 4 in]
        n145 = case shown="False" w351 {
          frame False {
            n146 = One Button Dialog(message="Some engineering parameters were missing") -> ()  [unwired: 1 in, 1 out]
          }
          frame True {
          }
        }
      }
      frame "READ_INI" {
        # "Read the configuration file and load the instrument state variables"
        n147 = global read "GSP_GUI_global.vi" "Configuration File"() -> (w364:path)
        n148 = call "Read_Master_Config.vi"("error in (no error)"=w358, "configuration file path"=w364) -> ("error out"=w357:errorcluster, "Present Configuration"=w359:T18)  [unwired: 3 in, 1 out]
        n149 = Unbundle By Name(w359) -> ("Primary Filter Names"=w360:string[], "Secondary Filter Names"=w361:string[], "Grating Names"=w362:string[], "Slit Mask Names"=w363:string[], "Standard Observing Modes"=w356:string[])
        n150 = global write "GSP_GUI_global.vi" "Standard Observing Mode Names"(w356) -> ()
        n151 = global write "GSP_GUI_global.vi" "Primary Filter Names"(w360) -> ()
        n152 = global write "GSP_GUI_global.vi" "Secondary Filter Names"(w361) -> ()
        n153 = global write "GSP_GUI_global.vi" "Slit Mask Names"(w363) -> ()
        n154 = global write "GSP_GUI_global.vi" "Grating Names"(w362) -> ()
      }
      frame "RESTART_SLIT" {
      }
      frame "SAVE_CONFIG" {
        n155 = call "GetSystemsInfo.vi"() -> ("Pos Info"=w381:T16)
        n156 = Unbundle By Name(w381) -> ("Camera Target"=w380:dbl, "Grating Target"=w379:dbl, "Coll Position"=w378:i32, "Camera Focus"=w377:i32)
        n157 = global read "GSP_GT_Global.vi" "Grating Name"() -> (w373:string)
        n158 = global read "GSP_SLIT_Global.vi" "Slit Name"() -> (w374:string)
        n159 = global read "GSP_F1_Global.vi" "F1_Name"() -> (w376:string)
        n160 = global read "GSP_F2_Global.vi" "F2_Name"() -> (w375:string)
        n161 = global read "GSP_Wavelength_Global.vi" "Flexure Active"() -> (w367:bool)
        n162 = Bundle("F1_Name"=w376, "F2_Name"=w375, "Slit Name"=w374, "Grating Name"=w373, "Camera Target"=w380, "Grating Target"=w379, "Coll Position"=w378, "Camera Focus"=w377, "", "", "", "", "Flexure Active"=w367, 0) -> (w372:T19)  [unwired: 1 in]
        n163 = call "SaveConfigGUI.vi"("error in (no error)"=w383, "Current Configuration"=w372) -> ("error out"=w382:errorcluster)  [unwired: 3 in, 2 out]
      }
      frame "SD_WAVELENGTH" {
        n164 = call "GSP_Manager_Wavelength_driver.vi"("error in (no error)"=w386, "Action"=wavelength_driver_actions."Shutdown") -> ("error out"=w385:errorcluster)  [unwired: 4 in, 1 out]
      }
      frame "SD_CF" {
        n165 = call "GSP_Manager_CF_driver.vi"("error in (no error)"=w389, "Action"=CF_drivercontrol."Shutdown") -> ("error out"=w388:errorcluster)  [unwired: 5 in, 1 out]
      }
      frame "SD_COLL" {
        n166 = call "GSP_Manager_COLL_driver.vi"("error in (no error)"=w391, "Action"=coll_actions."Shutdown") -> ("error out"=w392:errorcluster)  [unwired: 4 in, 1 out]
      }
      frame "SD_F1" {
        n167 = call "GSP_Manager_F1_driver.vi"("error in (no error)"=w395, "Action"=f1driveractions."Shutdown") -> ("error out"=w394:errorcluster)  [unwired: 4 in, 1 out]
      }
      frame "SD_F2" {
        n168 = call "GSP_Manager_F2_driver.vi"("error in (no error)"=w398, "Action"=f2driveractions."Shutdown") -> ("error out"=w397:errorcluster)  [unwired: 4 in, 1 out]
      }
      frame "SD_GT" {
        n169 = call "GSP_Manager_GT_driver.vi"("error in (no error)"=w401, "Action"=GTdriveractions."Shutdown") -> ("error out"=w400:errorcluster)  [unwired: 4 in, 1 out]
      }
      frame "SD_SLIT" {
        n170 = call "GSP_Manager_Slit_driver.vi"("error in (no error)"=w404, "Action"=slitactions."Shutdown") -> ("error out"=w403:errorcluster)  [unwired: 4 in, 1 out]
      }
      frame "SD_TCSLINK" {
        n171 = call "GSP_Manager_TCSLINK_handler.vi"("error in (no error)"=w407, "Actions"=TCSLINK_handler_actions."Shutdown") -> ("error out"=w406:errorcluster)  [unwired: 4 in, 1 out]
      }
      frame "SD_SICAMERA" {
        n172 = call "SIcamera_Driver.vi"("error in (no error)"=w409, "Action"=enum16{"Launch", "Shutdown"}."Shutdown") -> ("error out"=w408:errorcluster)  [unwired: 4 in, 1 out]
      }
      frame "SD_MODE" {
        n173 = call "Mode_driver.vi"("error in (no error)"=w413, "Action"=enum16{"Launch", "Shutdown"}."Shutdown") -> ("error out"=w412:errorcluster)  [unwired: 4 in, 1 out]
      }
      frame "SD_TCPSERVER" {
        n174 = call "TCPServer_driver.vi"("error in (no error)"=w416, "Action"=enum16{"Launch", "Shutdown"}."Shutdown") -> ("error out"=w415:errorcluster)  [unwired: 5 in]
      }
      frame "SD_SCLN" {
        n175 = flat-sequence {
          frame #0 {
            n176 = call "SCLN_SetShutdownFlagvi.vi"() -> ()  [unwired: 1 in]
          }
          frame #1 {
            n177 = Obtain Queue(name (unnamed)="SndToTCS_Command_Q", element data type="") -> (queue out=w418:refnum<queue>)  [unwired: 3 in, 2 out]
            n178 = Enqueue Element(queue=w418, element="WAY") -> ()  [unwired: 2 in, 3 out]
          }
        }
      }
      frame "SHOW_LOGGER" {
        n179 = call "GSP_Logger_Handler.vi"("error in (no error)"=w423, "Actions"=T4."Open") -> ("error out"=w421:errorcluster)  [unwired: 5 in]
      }
      frame "SHUTDOWN" {
        # "FINAL SHUDOWN - Release the queue and the port"
        n180 = Release Queue(queue=w425) -> ()  [unwired: 2 in, 3 out]
        n181 = call "gsp_silvermax_release.vi"() -> ("error out"=w424:errorcluster)  [unwired: 7 in]
      }
      frame "SLICER_IN" {
        n182 = Current VI's Menubar() -> (w434:refnum<k9>)
        n183 = Set Menu Item Info(7:"LOGOFF", 8:w432, 9:FALSE ("enabled"), 11:w434) -> (0:w429:errorcluster, 3:w430:refnum<k9>)  [unwired: 3 in]
        n184 = Set Menu Item Info(7:"USER", 8:w429, 9:FALSE ("enabled"), 11:w430) -> (0:w428:errorcluster)  [unwired: 3 in, 1 out]
      }
      frame "SLICER_OUT" {
        n185 = Current VI's Menubar() -> (w443:refnum<k9>)
        n186 = Set Menu Item Info(7:"LOGOFF", 8:w441, 9:TRUE ("enabled"), 11:w443) -> (0:w439:errorcluster, 3:w438:refnum<k9>)  [unwired: 3 in]
        n187 = Set Menu Item Info(7:"USER", 8:w439, 9:TRUE ("enabled"), 11:w438) -> (0:w436:errorcluster)  [unwired: 3 in, 1 out]
      }
      frame "WRITE_ENGINEERING" {
        n188 = global read "GSP_GUI_global.vi" "Engineering File"() -> (w446:path)
        n189 = call "Systems_WriteConfig.vi"("error in (no error)"=w445, "configuration file path"=w446) -> ("error out"=w444:errorcluster)  [unwired: 5 in]
      }
      frame "SHUTTER_CONTROL" {
        n190 = call "GSP_Shutter_ControlGUI.vi"("error in (no error)"=w448) -> ("error out"=w447:errorcluster)  [unwired: 6 in]
      }
      frame "WAIT_FOR_SHUTDOWN" {
        # "Use the Shutdown GUI to wait for all systems to shutdown before exiting."
        n191 = call "GUI_Shutdown.vi"("error in"=w449) -> ()  [unwired: 6 in, 1 out]
      }
    }
    n192 = Equal?(x=w14, y="SHUTDOWN") -> (x = y?=w12:bool)
    n193 = case shown="No Error" w8 {
      selector: w8 -> [_ w17]
      tunnel: w11 -> [_ w19]
      frame No Error {
      }
      frame Error {
        n194 = Enqueue Element At Opposite End(queue=w19, element="ERROR") -> ()  [unwired: 2 in, 3 out]
        "Last Error" <- w17
      }
    }
  }
